vi "mes初始化.vi"(10 "mes":string[][](array[string])) -> ()   [LabVIEW 2020]
uses:
  Global.vi
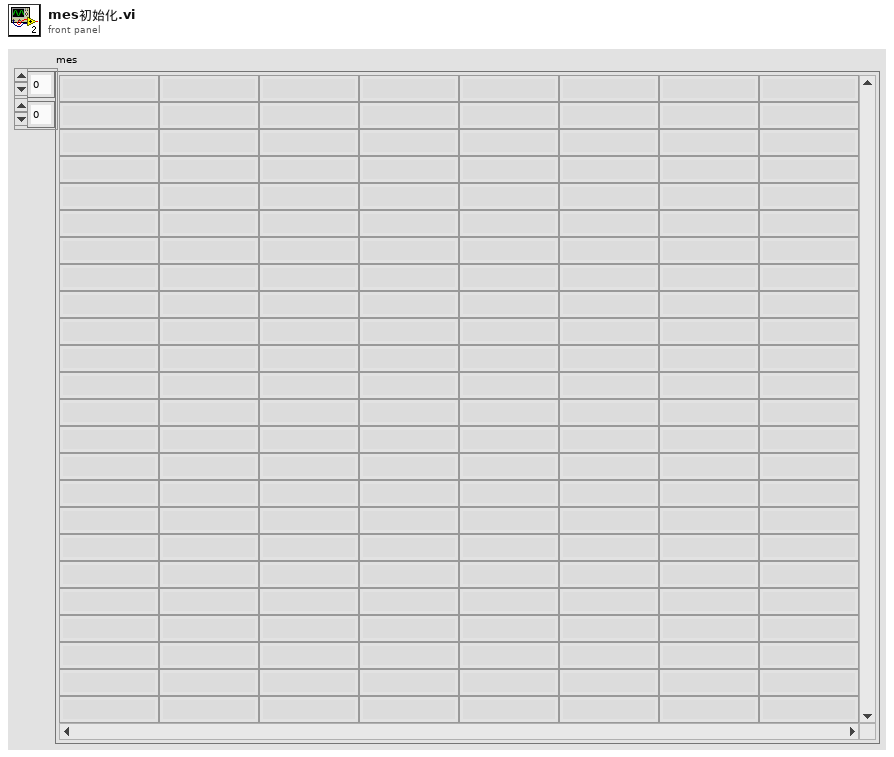
[diagram p1: front panel]
types:
  T1 = cluster{"接口地址(URL)":string, "用户登录":string, "产品进站":string, "数据上报":string, "产品出站":string, "设备状态":string, "设备编号(equipNum)":string, "站点名称(siteCode)":string, "生产类型(productType)":string, "试验单号(testOrderNum)":string}
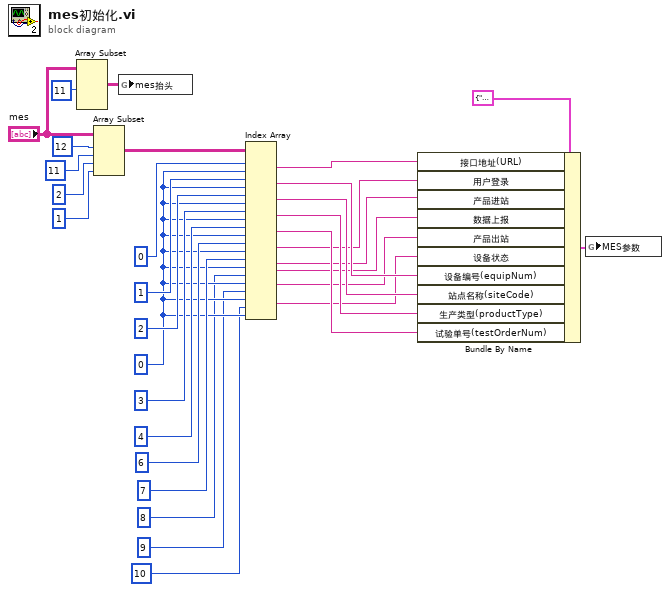
[diagram p0: block diagram]
diagram:
  w9 = 0 ("禁用的索引 (列)")
  n1 = Array Subset(array="mes", length (row)=11 ("索引 (行)")) -> (w27:string[][])  [unwired: 3 in]
  n2 = Array Subset(array="mes", index (row)=12 ("索引"), length (row)=11 ("长度"), index (col)=2 ("索引"), length (col)=1 ("长度")) -> (w24:string[][])
  n3 = global write "Global.vi" "mes抬头"(w27) -> ()
  n4 = Index Array(array=w24, index (row) #1=0 ("禁用的索引 (行)"), index (col) #1=w9, index (row) #2=1 ("禁用的索引 (列)"), index (col) #2=w9, index (row) #3=2 ("禁用的索引 (列)"), index (col) #3=w9, index (row) #4=3 ("禁用的索引 (列)"), index (col) #4=w9, index (row) #5=4 ("禁用的索引 (列)"), index (col) #5=w9, index (row) #6=6 ("禁用的索引 (列)"), index (col) #6=w9, index (row) #7=7 ("禁用的索引 (列)"), index (col) #7=w9, index (row) #8=8 ("禁用的索引 (列)"), index (col) #8=w9, index (row) #9=9 ("禁用的索引 (列)"), index (col) #9=w9, index (row) #10=10 ("禁用的索引 (列)"), index (col) #10=w9) -> (element #1=w18:string, element #2=w17:string, element #3=w16:string, element #4=w15:string, element #5=w14:string, element #6=w5:string, element #7=w4:string, element #8=w3:string, element #9=w2:string, element #10=w1:string)
  n5 = Bundle By Name(cluster=T1 {"接口地址(URL)"="", "用户登录"="", "产品进站"="", "数据上报"="", "产品出站"="", "设备状态"="", "设备编号(equipNum)"="", "站点名称(siteCode)"="", "生产类型(productType)"="", "试验单号(testOrderNum)"=""} ("MES参数"), "接口地址(URL)"=w18, "用户登录"=w5, "产品进站"=w4, "数据上报"=w3, "产品出站"=w2, "设备状态"=w1, "设备编号(equipNum)"=w17, "站点名称(siteCode)"=w16, "生产类型(productType)"=w15, "试验单号(testOrderNum)"=w14) -> (w13:T1)
  n6 = global write "Global.vi" "MES参数"(w13) -> ()
